vi "Get Convolution Product Support.vi"(8 "Error In":errorcluster, 9 "# Values":i32, 11 "IRF Period":dbl) -> (0 "Error Out":errorcluster, 1 "Step":dbl, 3 "Ramp":dbl[](array[numeric]))   [LabVIEW 2021, in "Fits.lvlib"]
uses:
  Fits.lvlib
  Arrays/Linear Ramp End Options.ctl
  ae4234dc-4024-40ff-b429-5ec38e02637d.vi
  6341dc52-b481-4549-9515-7aa03c41e646.vi
  3ac259e0-a0be-48f0-8a12-4717275a657e.vi
  Arrays/Arrays.lvlib
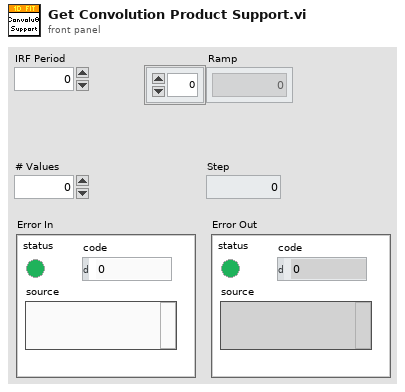
[diagram p1: front panel]
types:
  T1 = typedef "Arrays.lvlib/Linear Ramp End Options.ctl" = enum16{"Include Min/Exclude Max", "Exclude Min/Include Max", "Include Both Ends", "Exclude Both Ends"}
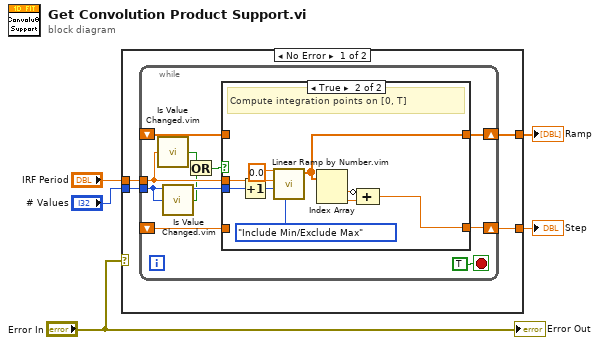
[diagram p0: block diagram]
diagram:
  n1 = case shown="No Error" "Error In" {
    tunnel: [w9 _] -> w5
    tunnel: [w8 _] -> w4
    tunnel: "# Values" -> [w7 _]
    tunnel: "IRF Period" -> [w6 _]
    frame No Error {
      n2 = while {
        tunnel: w6 -> [w13]
        tunnel: w7 -> [w12]
        shift-right: [w19] -> w8
        shift-left: _ -> [w17]
        shift-right: [w15] -> w9
        shift-left: _ -> [w14]
        stop <- TRUE stop-if-true
        n3 = call "Is Value Changed.vim"("value"=w13) -> ("changed or first call?"=w11:bool)
        n4 = call "Is Value Changed.vim"("value"=w12) -> ("changed or first call?"=w10:bool)
        n5 = Or(x=w11, y=w10) -> (x .or. y?=w16:bool)
        n6 = case shown="True" w16 {
          tunnel: [w20 w30] -> w15
          tunnel: [w21 w28] -> w19
          tunnel: w13 -> [_ w24]
          tunnel: w12 -> [_ w23]
          tunnel: w17 -> [w21 _]
          tunnel: w14 -> [w20 _]
          frame False {
            # "Use existing integration points"
          }
          frame True {
            # "Compute integration points on [0, T]"
            n7 = Increment(x=w23) -> (x+1=w22:i32)
            n8 = call "Linear Ramp by Number.vim"("Options"=Linear_Ramp_End_Options."Include Min/Exclude Max", "# Steps (1)"=w22, "End (1)"=w24, "Start (0)"=0.0) -> ("Ramp"=w28:dbl[])  [unwired: 5 in, 2 out]
            n9 = Index Array(array=w28) -> (element #1=w27:dbl, element #2=w29:dbl)  [unwired: 2 in]
            n10 = Compound Arithmetic op=ADD(invert w27, w29) -> (w30:dbl)
          }
        }
      }
    }
    frame Error {
    }
  }
  "Step" <- w5
  "Ramp" <- w4
  "Error Out" <- "Error In"
